vi "saveTestParameters.vi"(8 "error in (no error)":errorcluster, 11 "TestDataLog in":refnum<class "TestDataLog.lvclass">) -> (0 "error out":errorcluster, 3 "TestDataLog out":refnum<class "TestDataLog.lvclass">)   [LabVIEW 2013, in "TestDataLog.lvclass"]
uses:
  TestDataLog.lvclass
  <userlib>/Common/Log/Log/Log.lvclass
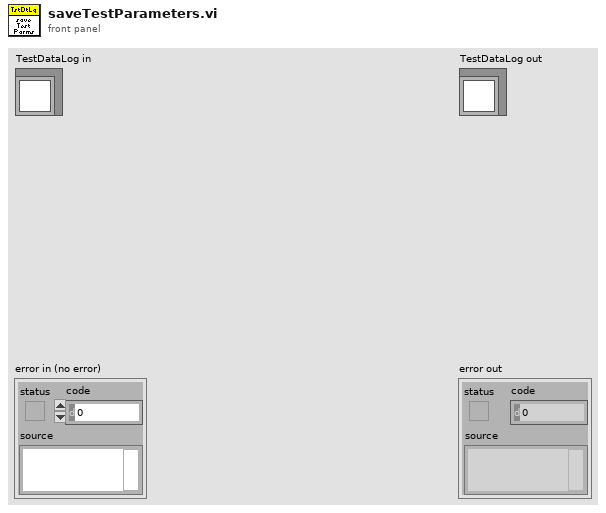
[diagram p1: front panel]
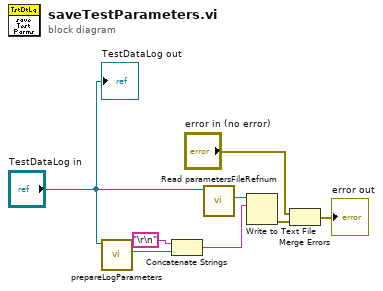
[diagram p0: block diagram]
diagram:
  n1 = call "prepareLogParameters.vi"("TestDataLog in"="TestDataLog in") -> ("LogParameters"=w3:string)  [unwired: 8 in, 2 out]
  n2 = Concatenate Strings("\r\n", w3) -> (w7:string)
  n3 = call <userlib>:"Read parametersFileRefnum.vi"("Log in"="TestDataLog in") -> ("parametersFileRefnum"=w8:refnum<file>)  [unwired: 9 in, 1 out]
  n4 = Write to Text File(file (use dialog)=w8, text=w7) -> (error out=w5:errorcluster)  [unwired: 2 in, 2 out]
  n5 = Merge Errors("error in (no error)", w5) -> (→"error out":errorcluster)
  "TestDataLog out" <- "TestDataLog in"
